vi "NISE.Connect.vi"(0 "SLSC Interface in":refnum<class "SLSC Interface.lvclass">, 5 "devices":refnum<k21>="$DefaultDevices", 11 "error in (no error)":errorcluster, 12 "connect timeout (60 sec)":dbl=60.0) -> (4 "SLSC Interface out":refnum<class "SLSC Interface.lvclass">, 15 "error out":errorcluster)   [LabVIEW 2016, in "SLSC Interface.lvclass"]
uses:
  SLSC Interface.lvclass
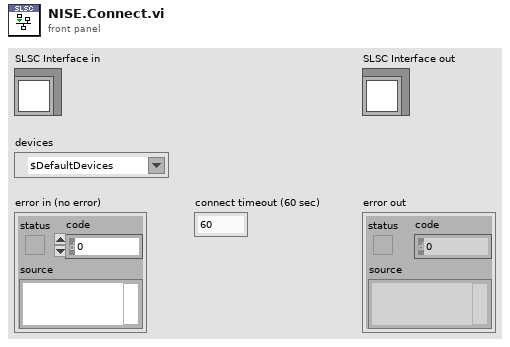
[diagram p1: front panel]
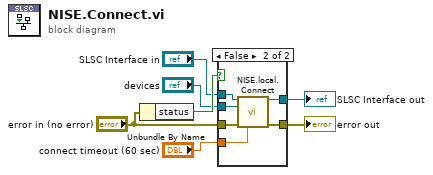
[diagram p0: block diagram]
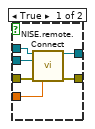
[diagram p2: hidden frame]
diagram:
  n1 = Unbundle By Name("error in (no error)") -> ("status"=w7:bool)
  n2 = case shown="False" w7 {
    tunnel: "SLSC Interface in" -> [w13 w19]
    tunnel: [w12 w18] -> w5
    tunnel: "devices" -> [w11 w17]
    tunnel: "error in (no error)" -> [w10 w16]
    tunnel: "connect timeout (60 sec)" -> [w9 w15]
    tunnel: [w8 w14] -> w1
    frame True {
      n3 = call "NISE.remote.Connect.vi"("SLSC Remote in"=w13, "devices"=w11, "error in (no error)"=w10, "connect timeout (60 sec)"=w9) -> ("SLSC Remote out"=w12:refnum<class "SLSC Interface.lvclass">, "error out"=w8:errorcluster)  [unwired: 10 in]
    }
    frame False {
      n4 = call "NISE.local.Connect.vi"("SLSC Local in"=w19, "devices"=w17, "error in (no error)"=w16, "connect timeout (60 sec)"=w15) -> ("SLSC Local out"=w18:refnum<class "SLSC Interface.lvclass">, "error out"=w14:errorcluster)  [unwired: 10 in]
    }
  }
  "error out" <- w1
  "SLSC Interface out" <- w5
